vi "Check_with_Jump_PN.vi"(0 "Current position":sgl[](array[numeric])=[0.0, 200.0, 40.0] format="%.2f", 1 "Traverse Name":string, 3 "Simulate/Run":T1=enum."Run VI", 5 "New Position":sgl[](array[numeric])=[0.0, 100.0, 40.0] format="%.2f", 14 "Model       Roll      Pitch       Yaw (deg)":sgl[](array[numeric]) format="%#.2f") -> (4 "Error Comments":string, 10 "Steps":sgl[][](array[numeric])=[[0.0, 200.0, 40.0]] format="%.2f")   [LabVIEW 2017]
uses:
  Route_mapping_global.vi
  Collision_Detection/Triangles/EnFlo specific/Collision Mode.ctl
  Controls/User_Specific_mode.ctl
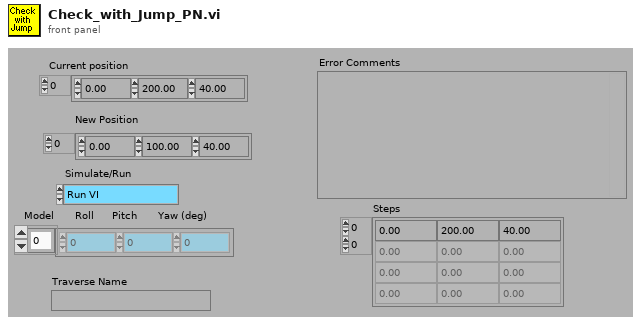
[diagram p1: front panel]
types:
  T1 = typedef "User_Specific_mode.ctl" = enum16{"Check VI only", "Run VI"}
  T2 = typedef "Box_size.ctl" = cluster{"Max":sgl, "Min":sgl}[]
  T3 = typedef "Collision Mode.ctl" = enum16{"Traverse - Tunnel", "Traverse - Model", "Traverse - Fixed objects", "Traverse - Traverse", "Traverse - All"}
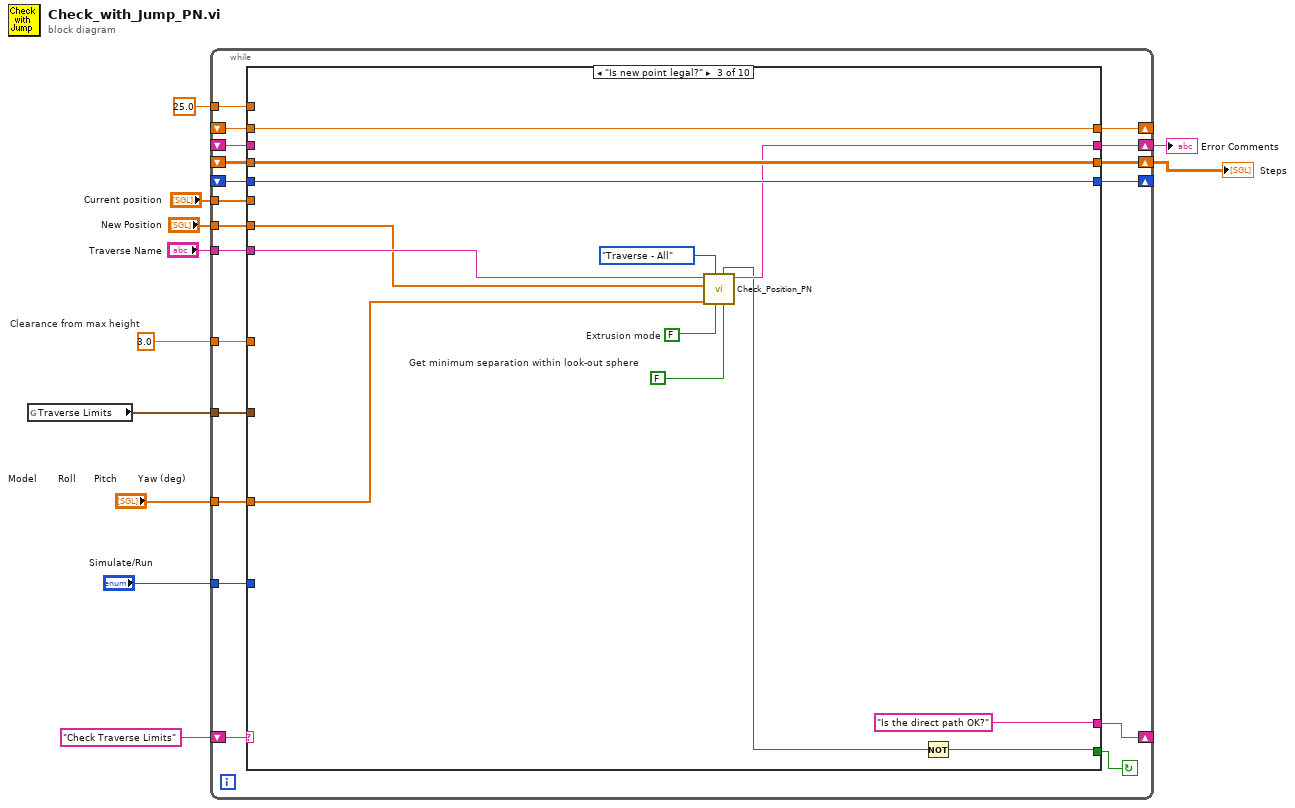
[diagram p0: block diagram]
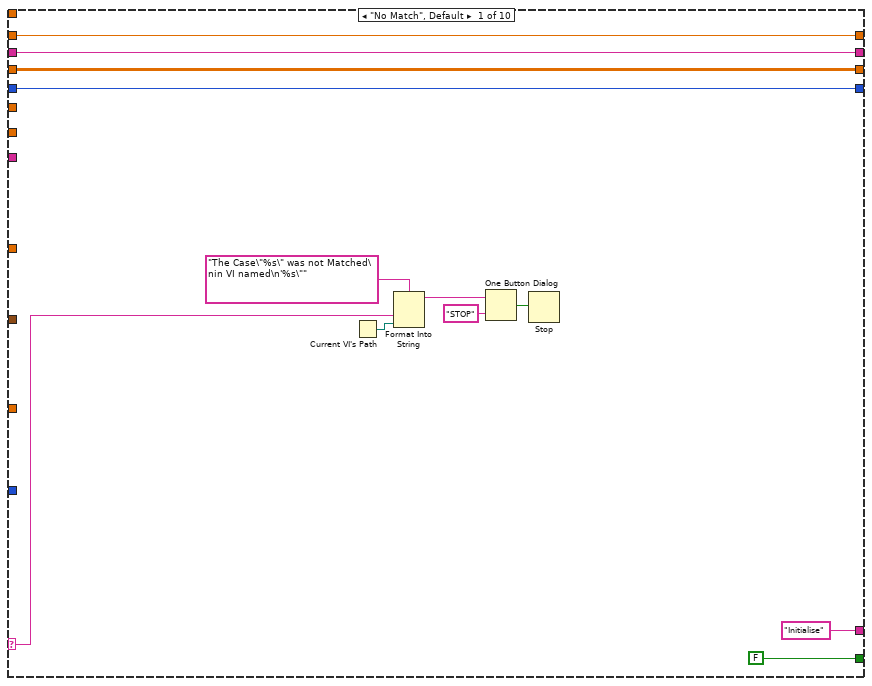
[diagram p2: hidden frame]
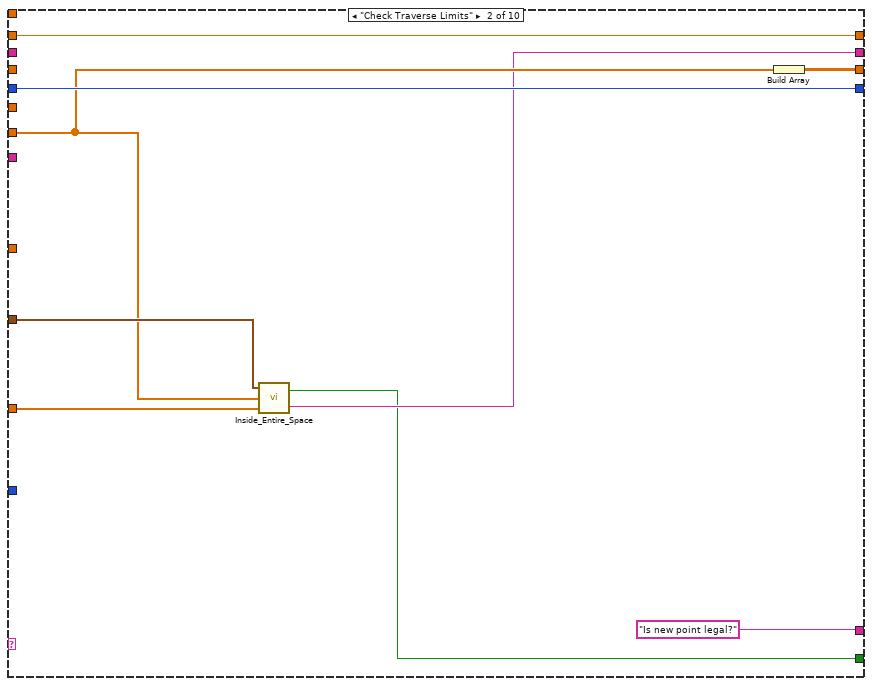
[diagram p3: hidden frame]
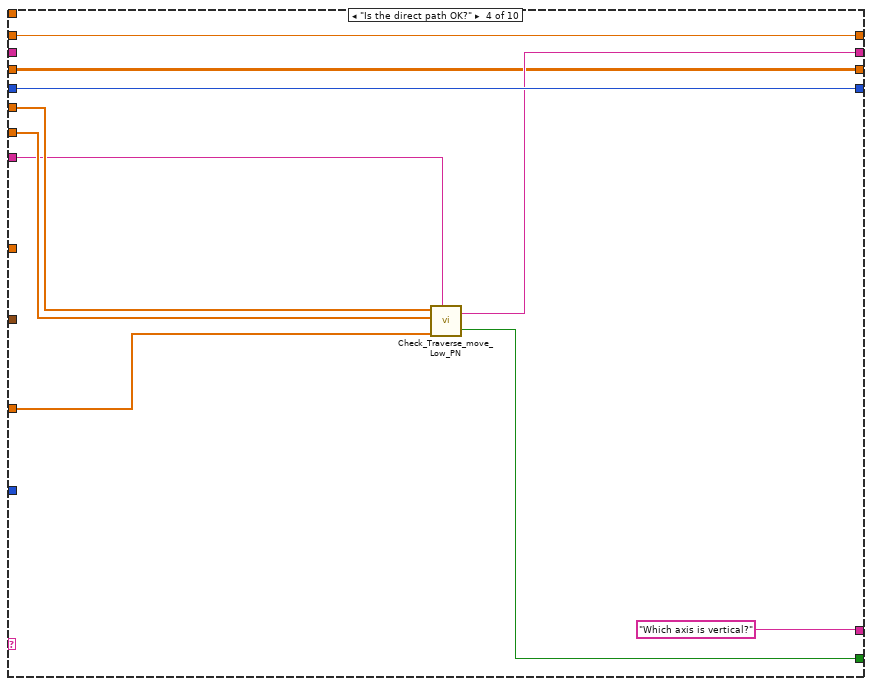
[diagram p4: hidden frame]
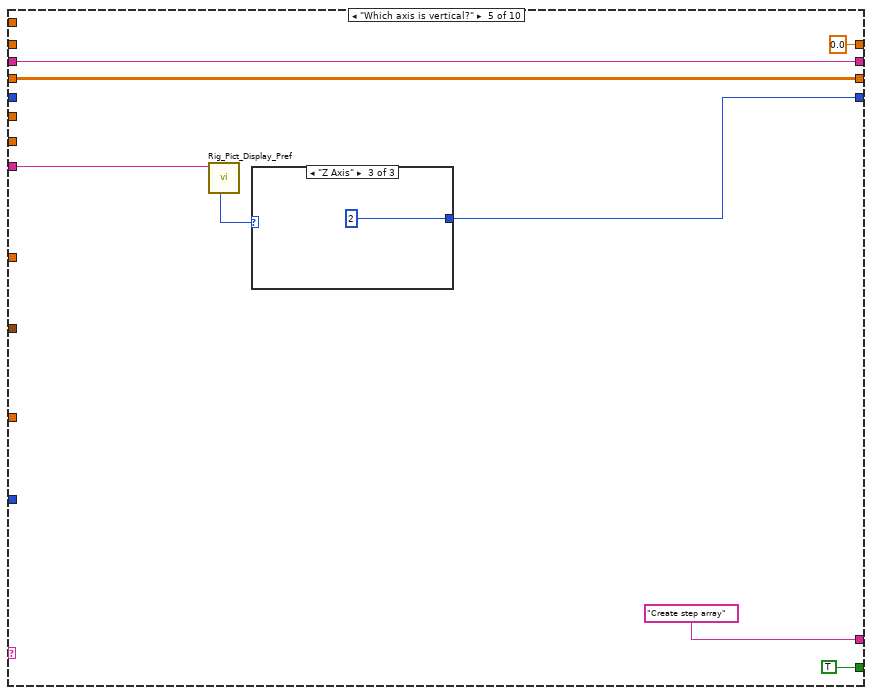
[diagram p5: hidden frame]
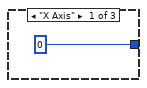
[diagram p6: hidden frame]
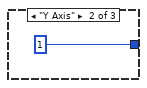
[diagram p7: hidden frame]
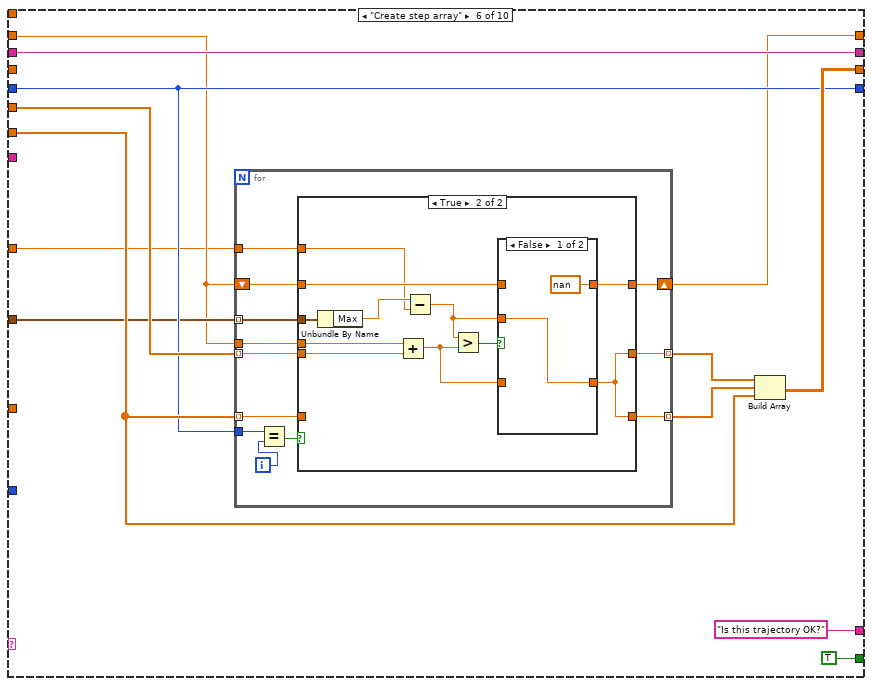
[diagram p8: hidden frame]
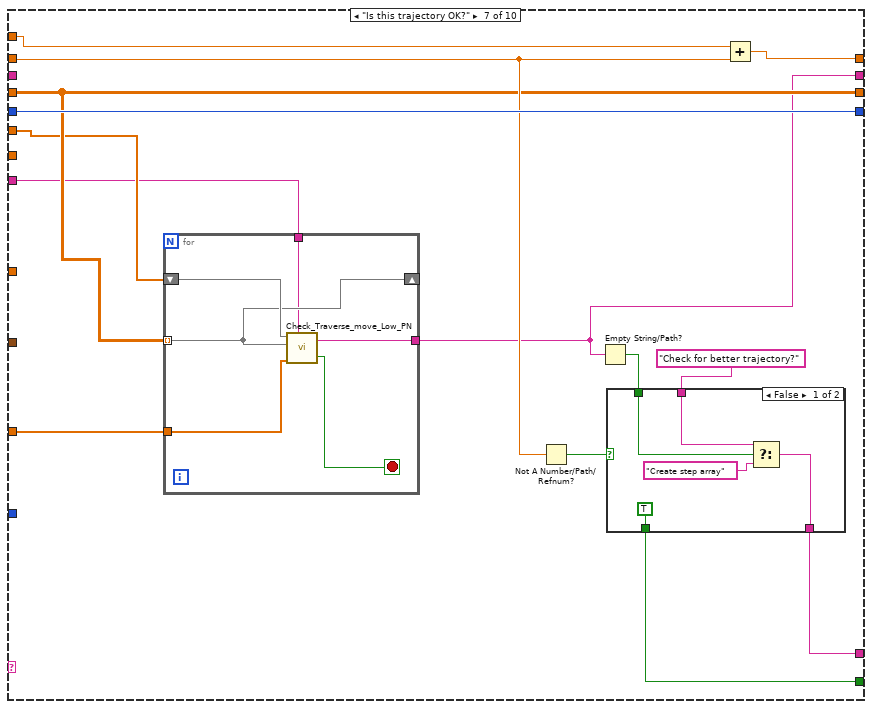
[diagram p11: hidden frame]
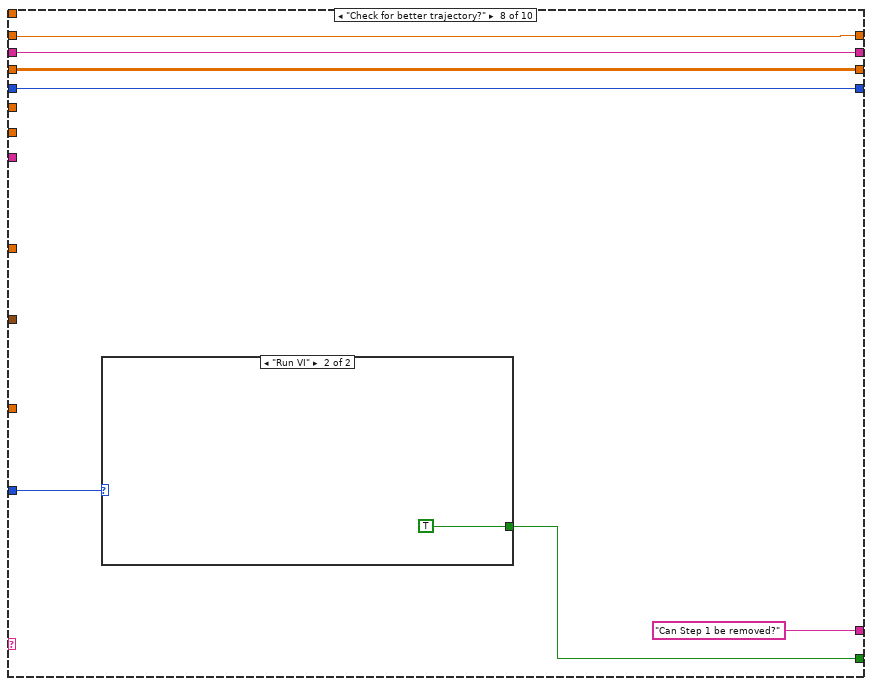
[diagram p13: hidden frame]
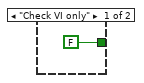
[diagram p14: hidden frame]
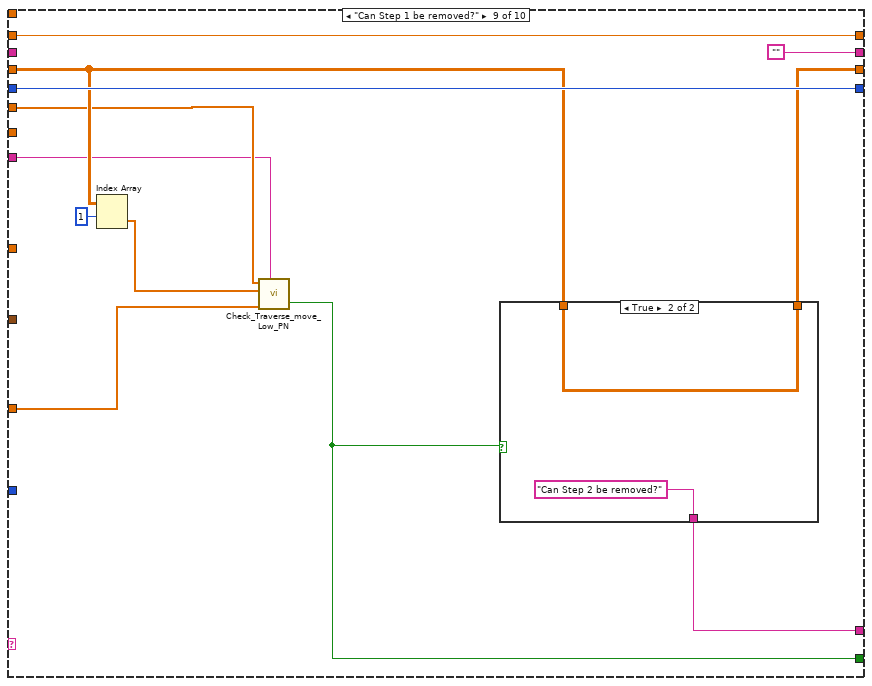
[diagram p15: hidden frame]
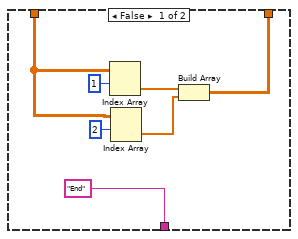
[diagram p16: hidden frame]
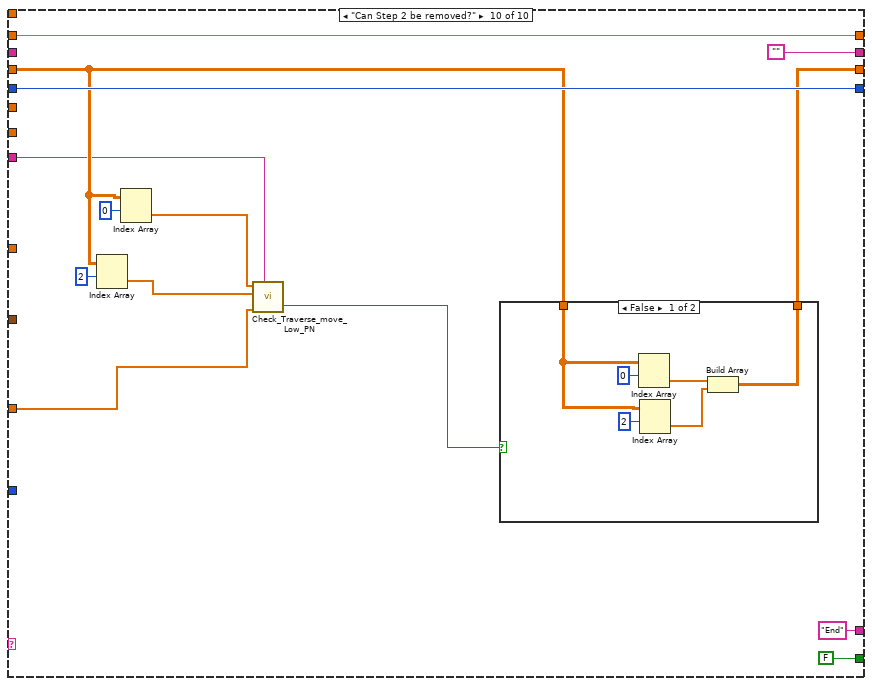
[diagram p17: hidden frame]
diagram:
  w1 = sgl 3.0  # Clearance from max height
  n1 = global read "Route_mapping_global.vi" "Traverse Limits"() -> (w2:T2)
  n2 = while {
    shift-left: "Check Traverse Limits" -> [w14]
    shift-right: [w30] -> _
    shift-right: [w27] -> w6
    shift-left: _ -> [w28]
    shift-right: [w26] -> w5
    shift-left: _ -> [w25]
    tunnel: "Current position" -> [w24]
    tunnel: "New Position" -> [w23]
    tunnel: "Traverse Name" -> [w22]
    shift-right: [w21] -> _
    shift-left: _ -> [w20]
    shift-right: [w19] -> _
    shift-left: _ -> [w18]
    tunnel: sgl 25.0 -> [w17]
    tunnel: "Simulate/Run" -> [w16]
    tunnel: "Model       Roll      Pitch       Yaw (deg)" -> [w15]
    tunnel: w2 -> [w13]
    tunnel: w1 -> [w12]
    stop <- w29 continue-if-true
    n3 = case shown="\"Is new point legal?\"" w14 {
      selector: w14 -> [w31 _ _ _ _ _ _ _ _ _]
      tunnel: [FALSE w43 w52 w66 TRUE TRUE w129 w156 w165 FALSE] -> w29
      tunnel: ["Initialise" "Is new point legal?" "Is the direct path OK?" "Which axis is vertical?" "Create step array" "Is this trajectory OK?" w140 "Can Step 1 be removed?" w170 "End"] -> w30
      tunnel: w28 -> [w35 _ _ _ w80 w97 _ w162 _ _]
      tunnel: [w35 w44 w54 w67 w80 w97 w130 w162 "" ""] -> w27
      tunnel: [w34 w48 w61 w65 w81 w91 w134 w159 w174 w197] -> w26
      tunnel: w25 -> [w34 _ w61 w65 w81 _ w134 w159 w173 w192]
      tunnel: w24 -> [_ _ _ w71 _ w95 w133 _ w169 _]
      tunnel: w23 -> [_ w45 w56 w70 _ w92 _ _ _ _]
      tunnel: w22 -> [_ _ w57 w68 w79 _ w131 _ w166 w188]
      tunnel: [w33 w50 w63 w73 w77 w90 w142 w161 w176 w199] -> w21
      tunnel: w20 -> [w33 w50 w63 w73 _ w90 w142 w161 w176 w199]
      tunnel: [w32 w51 w64 w74 sgl 0.0 w87 w138 w160 w172 w196] -> w19
      tunnel: w18 -> [w32 w51 w64 w74 _ w88 w137 w160 w172 w196]
      tunnel: w17 -> [_ _ _ _ _ _ w139 _ _ _]
      tunnel: w16 -> [_ _ _ _ _ _ _ w158 _ _]
      tunnel: w15 -> [_ w46 w55 w69 _ _ w132 _ w167 w189]
      tunnel: w13 -> [_ w47 _ _ _ w89 _ _ _ _]
      tunnel: w12 -> [_ _ _ _ _ w86 _ _ _ _]
      frame "No Match", Default {
        n4 = Current VI's Path() -> (path=w37:path)
        n5 = Format Into String(format string="The Case\"%s\" was not Matched\nin VI named\n'%s\"" ("Format String"), w31, w37) -> (resulting string=w40:string)  [unwired: 2 in, 1 out]
        n6 = One Button Dialog(message=w40, button name ("OK")="STOP") -> (true=w38:bool)
        n7 = Stop(stop? (T)=w38) -> ()
      }
      frame "Check Traverse Limits" {
        n8 = call "Inside_Entire_Space.vi"("Model       Roll      Pitch       Yaw (deg)"=w46, "Current Position"=w45, "Envelope"=w47) -> ("Error Comments"=w44:string, "Box Inside"=w43:bool)
        n9 = Build Array(w45) -> (w48:sgl[][])
      }
      frame "Is new point legal?" {
        w60 = FALSE  # Get minimum separation within look-out sphere
        w59 = FALSE  # Extrusion mode
        n10 = call "Check_Position_PN.vi"("Get minimum separation within look-out sphere"=w60, "Extrusion mode"=w59, "Collision mode"=Collision_Mode."Traverse - All", "Model Rotation (deg)"=w55, "Position to check"=w56, "Traverse Name"=w57) -> ("Error Comments"=w54:string, "Collision"=w53:bool)  [unwired: 2 in, 2 out]
        n11 = Not(x=w53) -> (.not. x?=w52:bool)
      }
      frame "Is the direct path OK?" {
        n12 = call "Check_Traverse_move_Low_PN.vi"("Current position"=w71, "New Position"=w70, "Model       Roll      Pitch       Yaw (deg)"=w69, "Traverse Name"=w68) -> ("Error Comments"=w67:string, "Collision"=w66:bool)  [unwired: 1 in]
      }
      frame "Which axis is vertical?" {
        n13 = call "Rig_Pict_Display_Pref.vi"("Traverse Name"=w79) -> ("Which Axis is vertical?"=w78:enum16{"X Axis", "Y Axis", "Z Axis"})  [unwired: 7 out]
        n14 = case shown="\"Z Axis\"" w78 {
          tunnel: [0 1 2] -> w77
          frame "X Axis" {
          }
          frame "Y Axis" {
          }
          frame "Z Axis" {
          }
        }
      }
      frame "Create step array" {
        n15 = for {
          tunnel: w88 -> [w110]
          tunnel: w90 -> [w107]
          tunnel: w95 -> [w106] mode=indexing
          tunnel: [w105] -> w94 mode=indexing
          tunnel: w92 -> [w104] mode=indexing
          tunnel: [w103] -> w93 mode=indexing
          tunnel: w89 -> [w102] mode=indexing
          shift-right: [w100] -> w87
          shift-left: w88 -> [w101]
          tunnel: w86 -> [w99]
          i -> [w109]
          n16 = Equal?(x=w107, y=w109) -> (x = y?=w108:bool)
          n17 = case shown="True" w108 {
            tunnel: w110 -> [_ w124]
            tunnel: w106 -> [w113 w123]
            tunnel: [w113 w120] -> w105
            tunnel: w104 -> [w112 _]
            tunnel: [w112 w120] -> w103
            tunnel: w102 -> [_ w122]
            tunnel: w101 -> [w111 w117]
            tunnel: [w111 w118] -> w100
            tunnel: w99 -> [_ w114]
            frame False {
            }
            frame True {
              n18 = Unbundle By Name(w122) -> ("Max"=w116:sgl)
              n19 = Add(x=w124, y=w123) -> (x+y=w119:sgl)
              n20 = Subtract(x=w116, y=w114) -> (x-y=w115:sgl)
              n21 = Greater?(x=w115, y=w119) -> (0:w121:bool)
              n22 = case shown="False" w121 {
                tunnel: [w125 w128] -> w120
                tunnel: w119 -> [_ w128]
                tunnel: [sgl nan w127] -> w118
                tunnel: w117 -> [_ w127]
                tunnel: w115 -> [w125 _]
                frame False {
                }
                frame True {
                }
              }
            }
          }
        }
        n23 = Build Array(w94, w93, w92) -> (w91:sgl[][])
      }
      frame "Is this trajectory OK?" {
        n24 = for {
          tunnel: w134 -> [w147] mode=indexing
          shift-right: [w147] -> _
          shift-left: w133 -> [w148]
          tunnel: w132 -> [w146]
          tunnel: w131 -> [w145]
          tunnel: [w143] -> w130
          stop <- w144 stop-if-true
          n25 = call "Check_Traverse_move_Low_PN.vi"("Current position"=w148, "New Position"=w147, "Model       Roll      Pitch       Yaw (deg)"=w146, "Traverse Name"=w145) -> ("Error Comments"=w143:string, "Collision"=w144:bool)  [unwired: 1 in]
        }
        n26 = Not A Number/Path/Refnum?(number/path/refnum=w137) -> (NaN/Path/Refnum?=w136:bool)
        n27 = Empty String/Path?(string/path=w130) -> (empty?=w141:bool)
        n28 = case shown="False" w136 {
          tunnel: w141 -> [w153 w154]
          tunnel: [w152 w155] -> w140
          tunnel: "Check for better trajectory?" -> [w150 w155]
          tunnel: [TRUE w154] -> w129
          frame False {
            n29 = Select(t=w150, s=w153, f="Create step array") -> (s? t:f=w152:string)
          }
          frame True {
          }
        }
        n30 = Add(x=w139, y=w137) -> (x+y=w138:sgl)
      }
      frame "Check for better trajectory?" {
        n31 = case shown="\"Run VI\"" w158 {
          tunnel: [FALSE TRUE] -> w156
          frame "Check VI only" {
          }
          frame "Run VI" {
          }
        }
      }
      frame "Can Step 1 be removed?" {
        n32 = Index Array(array=w173, index (row)=1) -> (element=w168:sgl[])  [unwired: 1 in]
        n33 = call "Check_Traverse_move_Low_PN.vi"("Current position"=w169, "New Position"=w168, "Model       Roll      Pitch       Yaw (deg)"=w167, "Traverse Name"=w166) -> ("Collision"=w165:bool)  [unwired: 1 in, 1 out]
        n34 = case shown="True" w165 {
          tunnel: [w178 w185] -> w174
          tunnel: w173 -> [w181 w185]
          tunnel: ["End" "Can Step 2 be removed?"] -> w170
          frame False {
            n35 = Index Array(array=w181, index (row)=1) -> (element=w180:sgl[])  [unwired: 1 in]
            n36 = Index Array(array=w181, index (row)=2) -> (element=w179:sgl[])  [unwired: 1 in]
            n37 = Build Array(w180, w179) -> (w178:sgl[][])
          }
          frame True {
          }
        }
      }
      frame "Can Step 2 be removed?" {
        n38 = Index Array(array=w192, index (row)=2) -> (element=w190:sgl[])  [unwired: 1 in]
        n39 = Index Array(array=w192, index (row)=0) -> (element=w191:sgl[])  [unwired: 1 in]
        n40 = call "Check_Traverse_move_Low_PN.vi"("Current position"=w191, "New Position"=w190, "Model       Roll      Pitch       Yaw (deg)"=w189, "Traverse Name"=w188) -> ("Collision"=w187:bool)  [unwired: 1 in, 1 out]
        n41 = case shown="False" w187 {
          tunnel: [w200 w206] -> w197
          tunnel: w192 -> [w203 w206]
          frame False {
            n42 = Index Array(array=w203, index (row)=0) -> (element=w202:sgl[])  [unwired: 1 in]
            n43 = Index Array(array=w203, index (row)=2) -> (element=w201:sgl[])  [unwired: 1 in]
            n44 = Build Array(w202, w201) -> (w200:sgl[][])
          }
          frame True {
          }
        }
      }
    }
  }
  "Error Comments" <- w6
  "Steps" <- w5
